vi "Load DQMH Modules From Project.vi"(6 "TreeControl in":refnum<vi>, 7 "Data Cluster In":T1, 8 "error in":errorcluster, 11 "Project Path":path=path "C:/Users/Enrique Noé Arias/Desktop/Untitled Project 1/PantherScan.xml") -> (0 "error out":errorcluster, 5 "Data Cluster Out":T1={"DQMH Scan Results"={"All DQMH Modules Refs"=[], "All Modules Descriptions"=[], "All Modules type"=[], "Project References"={"Project Ref"=refnum, "Project Name"="", "Target"=refnum, "App Ref"=refnum}, "Dependencies"=[]}, "Current Selection"={"VI Ref"=refnum, "DQMH Lib Ref"=refnum}, "Module type"=enum."Singleton", "Module ID"=-1, "Theme"=FALSE, "Broadcast?"=FALSE, "Tree Selection"="", "Tree Map"={}})   [LabVIEW 2019, in "Panther Dashboard.lvlib"]
doc: "Gets the Singleton and Cloneable references and creates a list of each type of DQMH Modules"
uses:
  Panther Dashboard.lvlib
  Module Data--cluster.ctl
  DQMH Modules Info--cluster.ctl
  Module type--enum.ctl
  Project References--cluster.ctl
  <vilib>/National Instruments/Tree Map/Tree Map Data.ctl
  <vilib>/National Instruments/Tree Map/API/List Roots.vi
  <vilib>/National Instruments/Tree Map/Utility/Into Tree Control Items.vi
  <vilib>/National Instruments/Tree Map/Tree Map.lvlib
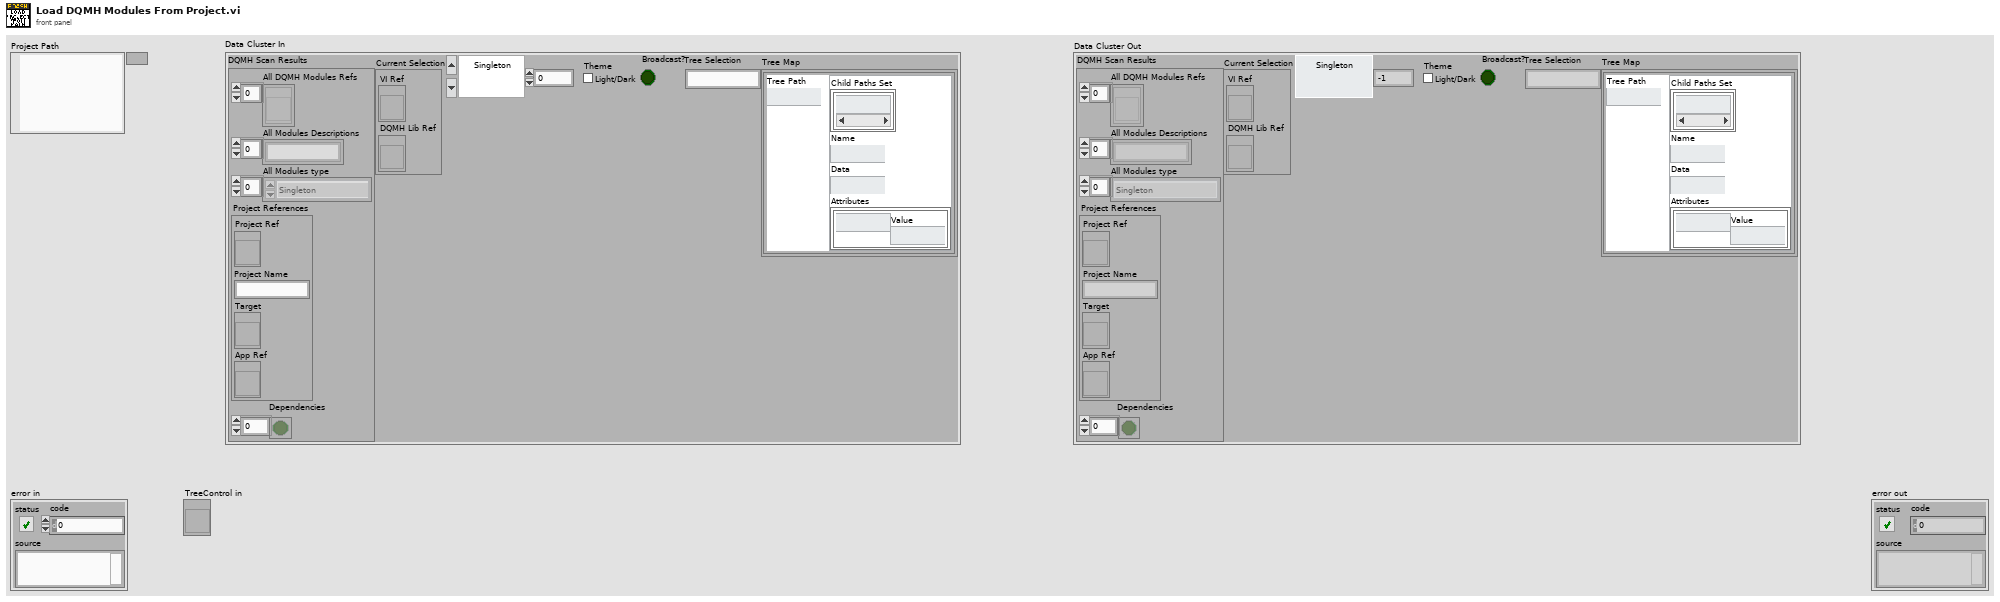
[diagram p1: front panel]
types:
  T1 = typedef "Panther Dashboard.lvlib/Module Data--cluster.ctl" = cluster{"DQMH Scan Results":T2, "Current Selection":cluster{"VI Ref":refnum<vi>, "DQMH Lib Ref":refnum<vi>}, "Module type":T3, "Module ID":i32, "Theme":bool, "Broadcast?":bool, "Tree Selection":string, "Tree Map":T5}
  T2 = typedef "Panther Dashboard.lvlib/DQMH Modules Info--cluster.ctl" = cluster{"All DQMH Modules Refs":refnum<vi>[], "All Modules Descriptions":string[], "All Modules type":T3[], "Project References":T4, "Dependencies":bool[]}
  T3 = typedef "Panther Dashboard.lvlib/Module type--enum.ctl" = enum16{"Singleton", "Cloneable"}
  T4 = typedef "Panther Dashboard.lvlib/Project References--cluster.ctl" = cluster{"Project Ref":refnum<vi>, "Project Name":string, "Target":refnum<vi>, "App Ref":refnum<vi>}
  T5 = typedef "Tree Map.lvlib/Tree Map Data.ctl" = map{string, cluster{"Child Paths Set":set{string}, "Name":string, "Data":string, "Attributes":map{string, string}}}
  T6 = cluster{"Left Cell String":string, "Child Text":string[], "Child Tag":string, "Item Indent":i32, "Child Only?":bool, "Glyph Index":i32}[]
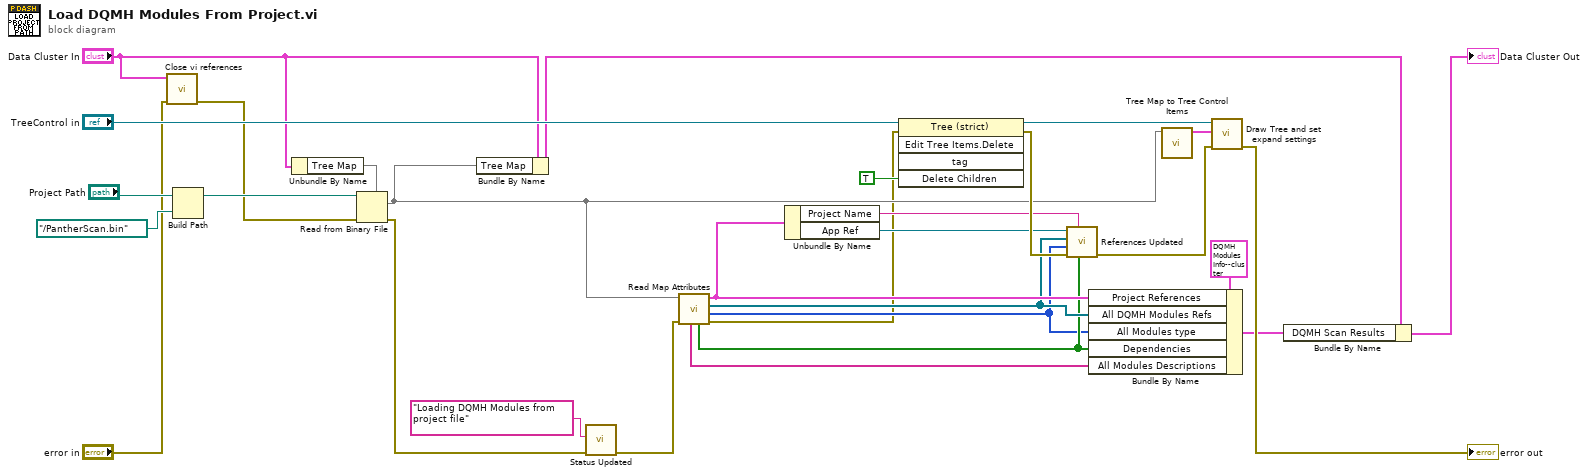
[diagram p0: block diagram]
diagram:
  n1 = call "Close vi references.vi"("error in"="error in", "Data Cluster"="Data Cluster In") -> ("error out"=w1:errorcluster)  [unwired: 9 in]
  n2 = Build Path(base path="Project Path", name or relative path=path "../PantherScan.bin") -> (appended path=w12:path)
  n3 = Unbundle By Name("Data Cluster In") -> ("Tree Map"=w5:T5)
  n4 = Read from Binary File(5:w5, 8:w1, 11:w12) -> (0:w29:errorcluster, 2:w19:T5)  [unwired: 3 in, 2 out]
  n5 = Bundle By Name(cluster="Data Cluster In", "Tree Map"=w19) -> (w22:T1)
  n6 = call "Status Updated.vi"("error in (no error)"=w29, "Status"="Loading DQMH Modules from project file") -> ("error out"=w6:errorcluster)  [unwired: 9 in]
  n7 = call "Read Map Attributes.vi"("error in"=w6, "Tree Map In (empty)"=w19) -> ("error out"=w3:errorcluster, "Modules Types Out"=w8:T3[], "Library References"=w20:refnum<vi>[], "References"=w21:T4, "Dependencies?"=w9:bool[], "Descriptions"=w10:string[])  [unwired: 4 in]
  n8 = Unbundle By Name(w21) -> ("Project Name"=w13:string, "App Ref"=w7:refnum<vi>)
  n9 = invoke class="Tree (strict)" method="Edit Tree Items.Delete"(reference="TreeControl in", error in=w3, "Delete Children"=TRUE ("Delete Children?")) -> (reference out=w14:refnum<vi>, error out=w28:errorcluster)  [unwired: 2 in, 3 out]
  n10 = call "References Updated.vi"("Dependencies"=w9, "Project Name"=w13, "error in"=w28, "Modules Types"=w8, "Modules"=w20, "Application Instance"=w7) -> ("error out"=w27:errorcluster)  [unwired: 5 in]
  n11 = Bundle By Name(cluster=T2 {"All DQMH Modules Refs"=[], "All Modules Descriptions"=[], "All Modules type"=[], "Project References"={"Project Ref"=refnum, "Project Name"="", "Target"=refnum, "App Ref"=refnum}, "Dependencies"=[]} ("DQMH Scan Results"), "Project References"=w21, "All DQMH Modules Refs"=w20, "All Modules type"=w8, "Dependencies"=w9, "All Modules Descriptions"=w10) -> (w17:T2)
  n12 = call <vilib>:"Tree Map to Tree Control Items.vi"("Tree Map In"=w19) -> ("Tree Control Items"=w16:T6)  [unwired: 10 in]
  n13 = call "Draw Tree and set expand settings.vi"("error in"=w27, "Tree Control Items"=w16, "TreeControl in"=w14) -> ("error out"=→"error out":errorcluster)  [unwired: 8 in]
  n14 = Bundle By Name(cluster=w22, "DQMH Scan Results"=w17) -> (→"Data Cluster Out":T1)
